vi "DeCoF FilterCommandError.vi"(5 "error in (no error)":errorcluster) -> (1 "error out":errorcluster, 2 "command error?":bool)   [LabVIEW 2013]
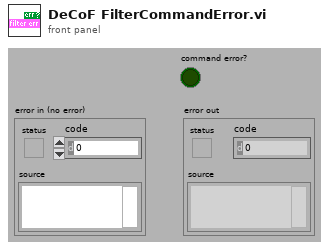
[diagram p1: front panel]
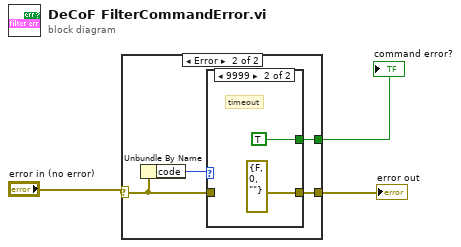
[diagram p0: block diagram]
diagram:
  n1 = case shown="Error" "error in (no error)" {
    selector: "error in (no error)" -> [w4 w8]
    tunnel: [w4 w6] -> w2
    tunnel: [_ w5] -> w1
    frame No Error {
    }
    frame Error {
      n2 = Unbundle By Name(w8) -> ("code"=w7:i32)
      n3 = case shown="9999" w7 {
        tunnel: w8 -> [w9 _]
        tunnel: [w9 errorcluster {"status"=FALSE, "code"=0, "source"=""} ("error IO")] -> w6
        tunnel: [_ TRUE] -> w5
        frame 0, Default {
        }
        frame 9999 {
          # "timeout"
        }
      }
    }
  }
  "error out" <- w2
  "command error?" <- w1
